vi "Extend Display Range to Match Slider(s).vi"(8 "error in (no error)":errorcluster, 11 "Display Range":refnum<vi>) -> (0 "error out":errorcluster, 1 "Range Min Updated":bool, 2 "Range Max Updated":bool)   [LabVIEW 2021, in "GUI.lvlib"]
doc: "If the sliders are outside the displayed range, extend the displayed range."
uses:
  GUI.lvlib
panel:
  # "see the AlliGator License on the block diagram (Ctrl+E or Window:Show Block Diagram)"
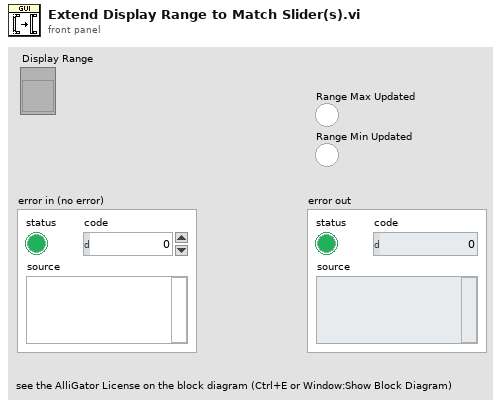
[diagram p1: front panel]
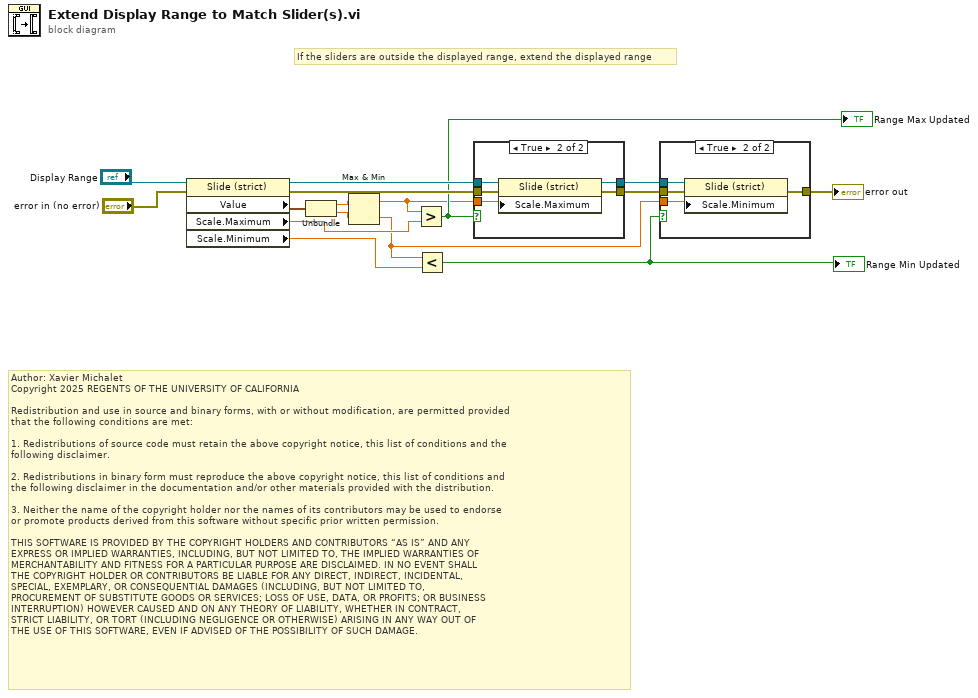
[diagram p0: block diagram]
diagram:
  # "If the sliders are outside the displayed range, extend the displayed range"
  # "Author: Xavier Michalet\nCopyright 2025 REGENTS OF THE UNIVERSITY OF CALIFORNIA\n\nRedistribution and use in source and binary forms, with or without modification, are permitted provided\nthat the following conditions are met:\n\n1. Redistributions of source code must retain the above copyright notice, this list of conditions and the\nfollowing disclaimer.\n\n2. Redistributions in binary form must reproduce the above copyright notice, this list of conditions and\nthe following disclaimer in the documentation and/or other materials provided with the distribution.\n\n3. Neither the name of the copyright holder nor the names of its contributors may be used to endorse \nor promote products derived from this software without specific prior written permission.\n\nTHIS SOFTWARE IS PROVIDED BY THE COPYRIGHT HOLDERS AND CONTRIBUTORS “AS IS” AND ANY \nEXPRESS OR IMPLIED WARRANTIES, INCLUDING, BUT NOT LIMITED TO, THE IMPLIED WARRANTIES OF\nMERCHANTABILITY AND FITNESS FOR A PARTICULAR PURPOSE ARE DISCLAIMED. IN NO EVENT SHALL\nTHE COPYRIGHT HOLDER OR CONTRIBUTORS BE LIABLE FOR ANY DIRECT, INDIRECT, INCIDENTAL, \nSPECIAL, EXEMPLARY, OR CONSEQUENTIAL DAMAGES (INCLUDING, BUT NOT LIMITED TO, \nPROCUREMENT OF SUBSTITUTE GOODS OR SERVICES; LOSS OF USE, DATA, OR PROFITS; OR BUSINESS\nINTERRUPTION) HOWEVER CAUSED AND ON ANY THEORY OF LIABILITY, WHETHER IN CONTRACT, \nSTRICT LIABILITY, OR TORT (INCLUDING NEGLIGENCE OR OTHERWISE) ARISING IN ANY WAY OUT OF\nTHE USE OF THIS SOFTWARE, EVEN IF ADVISED OF THE POSSIBILITY OF SUCH DAMAGE."
  n1 = property class="Slide (strict)"(reference="Display Range", error in="error in (no error)") -> (reference out=w12:refnum<vi>, error out=w11:errorcluster, "Value"=w15:cluster{dbl, dbl}, "Scale.Maximum"=w9:dbl, "Scale.Minimum"=w6:dbl)
  n2 = Unbundle(w15) -> (w14:dbl, w13:dbl)
  n3 = Max & Min(x=w14, y=w13) -> (max(x,y)=w7:dbl, min(x,y)=w3:dbl)
  n4 = Greater?(x=w7, y=w9) -> (0:w8:bool)
  "Range Max Updated" <- w8
  n5 = Less?(x=w3, y=w6) -> (x < y?=w1:bool)
  "Range Min Updated" <- w1
  n6 = case shown="True" w8 {
    tunnel: w12 -> [w18 w23]
    tunnel: w11 -> [w17 w22]
    tunnel: w7 -> [_ w21]
    tunnel: [w18 w20] -> w5
    tunnel: [w17 w19] -> w4
    frame False {
    }
    frame True {
      n7 = property class="Slide (strict)"(reference=w23, error in=w22, "Scale.Maximum"=w21) -> (reference out=w20:refnum<vi>, error out=w19:errorcluster)
    }
  }
  n8 = case shown="True" w1 {
    tunnel: w5 -> [_ w28]
    tunnel: w4 -> [w24 w27]
    tunnel: w3 -> [_ w26]
    tunnel: [w24 w25] -> w2
    frame False {
    }
    frame True {
      n9 = property class="Slide (strict)"(reference=w28, error in=w27, "Scale.Minimum"=w26) -> (error out=w25:errorcluster)  [unwired: 1 out]
    }
  }
  "error out" <- w2
